vi "UnitTest-Initialize.vi"(8 "error in":errorcluster, 11 "Config IN":T2={"TableLogger"=enum."CSV Logger", "DB File Path"=path "C:/FD/Test.csv", "DB Backup Config"={"Directory"=path "C:/LogAnyLVdata", "UTC Time Format"=FALSE, "On Launch"=TRUE, "Interval (Hours)"=100.0, "Size Multiples (Bytes)"=24}}) -> (0 "error out":errorcluster, 2 "LV Data":T1={"Numeric Data"=1, "Float Data"=1.0, "String Data"="This is string", "Enum Data"=enum."Enum Item 2", "Array Data"=[1234, 2345, 3456, 4567]}, 3 "Config OUT":T2={"TableLogger"=enum."SQLite Logger", "DB File Path"=path "DB.db", "DB Backup Config"={"Directory"=path "DB/Backup", "UTC Time Format"=FALSE, "On Launch"=FALSE, "Interval (Hours)"=100.0, "Size Multiples (Bytes)"=24}})   [LabVIEW 2014]
uses:
  TableLogger_Actor/TableLoggerConfig.ctl
  TableLogger_Actor/TableLoggerTypes.ctl
  TableLogger_Actor/TableLoggerBackupConfig.ctl
  TableLogger_Actor/TableLoggerDataCluster.ctl
  <userlib>/_OpenG.lib/file/file.llb/Strip Path - Traditional__ogtk.vi
  <userlib>/_OpenG.lib/file/file.llb/File Exists - Scalar__ogtk.vi
  <userlib>/_OpenG.lib/file/file.llb/Build Path - Traditional__ogtk.vi
  TableLogger_Actor/TableLogger_Actor.lvlib
panel:
  # "Connector Pane"
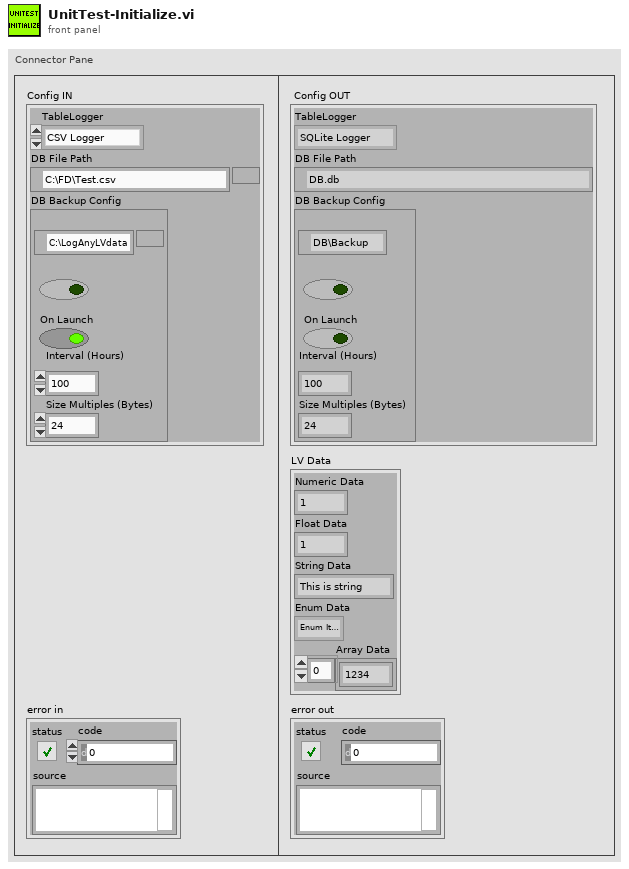
[diagram p1: front panel]
types:
  T1 = typedef "TableLogger_Actor.lvlib/TableLoggerDataCluster.ctl" = cluster{"Numeric Data":i32, "Float Data":dbl, "String Data":string, "Enum Data":enum16{"Enum Item 1", "Enum Item 2"}, "Array Data":i32[]}
  T2 = typedef "TableLogger_Actor.lvlib/TableLoggerConfig.ctl" = cluster{"TableLogger":T3, "DB File Path":path, "DB Backup Config":T4}
  T3 = typedef "TableLogger_Actor.lvlib/TableLoggerTypes.ctl" = enum16{"CSV Logger", "SQLite Logger"}
  T4 = typedef "TableLogger_Actor.lvlib/TableLoggerBackupConfig.ctl" = cluster{"Directory":path, "UTC Time Format":bool, "On Launch":bool, "Interval (Hours)":dbl, "Size Multiples (Bytes)":i32}
  T5 = enum16{"open", "replace", "create", "open or create", "replace or create", "replace or create with confirmation"}
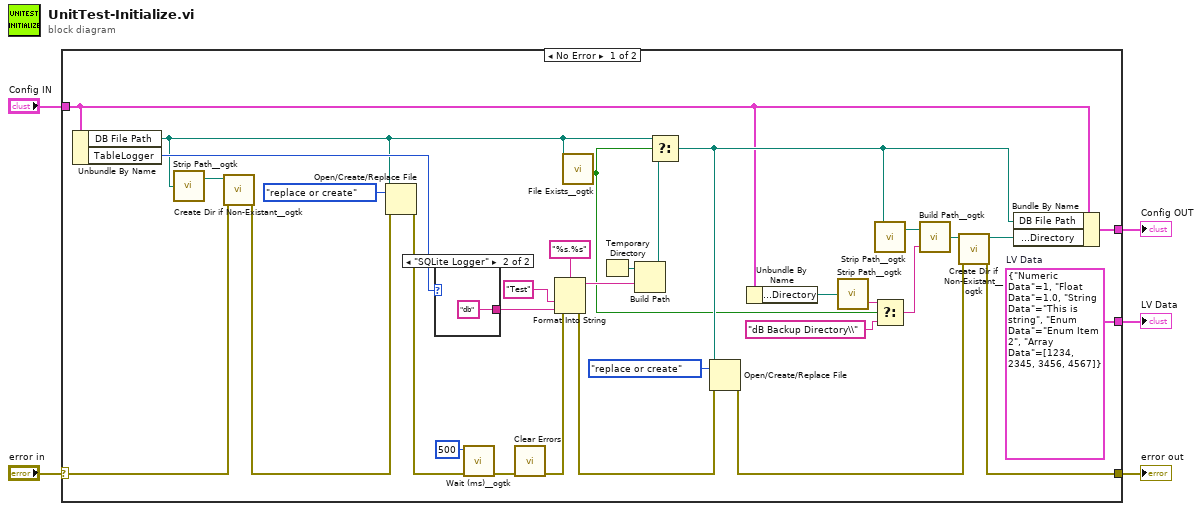
[diagram p0: block diagram]
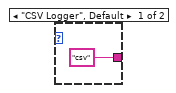
[diagram p2: hidden frame]
diagram:
  n1 = case shown="No Error" "error in" {
    selector: "error in" -> [w8 w41]
    tunnel: [w26 w41] -> w4
    tunnel: "Config IN" -> [w13 w40]
    tunnel: [w34 w40] -> w2
    tunnel: [w6 _] -> w1
    frame No Error {
      w6 = T1 {"Numeric Data"=1, "Float Data"=1.0, "String Data"="This is string", "Enum Data"=enum."Enum Item 2", "Array Data"=[1234, 2345, 3456, 4567]}  # LV Data
      n2 = Unbundle By Name(w13) -> ("DB File Path"=w10:path, "TableLogger"=w33:T3)
      n3 = call-poly <userlib>:"Strip Path__ogtk.vi"("path"=w10) -> ("stripped path"=w9:path)  [unwired: 1 out]
      n4 = call <userlib>:"Create Dir if Non-Existant__ogtk.vi"("error in (no error)"=w8, "Directory Path"=w9) -> ("error out"=w7:errorcluster)  [unwired: 7 in, 2 out]
      n5 = Open/Create/Replace File(file path (use dialog)=w10, error in=w7, operation (0:open)=T5."replace or create") -> (error out=w12:errorcluster)  [unwired: 3 in, 2 out]
      n6 = case shown="\"SQLite Logger\"" w33 {
        tunnel: ["csv" ("format string") "db" ("format string")] -> w32
        frame "CSV Logger", Default {
        }
        frame "SQLite Logger" {
        }
      }
      n7 = call <userlib>:"Wait (ms)__ogtk.vi"("error in (no error)"=w12, "milliseconds to wait"=u32 500) -> ("error out"=w21:errorcluster)  [unwired: 8 in, 1 out]
      n8 = call <vilib>:"Clear Errors.vi"("error in (no error)"=w21) -> ("error out"=w11:errorcluster)  [unwired: 5 in, 1 out]
      n9 = Format Into String(format string="%s.%s", error in=w11, "Test" ("input 1"), w32) -> (resulting string=w35:string, error out=w19:errorcluster)  [unwired: 1 in]
      n10 = call-poly <userlib>:"File Exists__ogtk.vi"("file path"=w10) -> ("exists"=w18:bool)  [unwired: 6 in, 1 out]
      n11 = Temporary Directory() -> (w37:path)
      n12 = Build Path(base path=w37, name or relative path=w35) -> (appended path=w30:path)
      n13 = Select(t=w10, s=w18, f=w30) -> (s? t:f=w25:path)
      n14 = Open/Create/Replace File(file path (use dialog)=w25, error in=w19, operation (0:open)=T5."replace or create") -> (error out=w24:errorcluster)  [unwired: 3 in, 2 out]
      n15 = Unbundle By Name(w13) -> ("DB Backup Config.Directory"=w14:path)
      n16 = call-poly <userlib>:"Strip Path__ogtk.vi"("path"=w14) -> ("name"=w15:string)  [unwired: 1 out]
      n17 = call-poly <userlib>:"Strip Path__ogtk.vi"("path"=w25) -> ("stripped path"=w29:path)  [unwired: 1 out]
      n18 = Select(t=w15, s=w18, f="dB Backup Directory\\" ("name or relative path")) -> (s? t:f=w16:string)
      n19 = call-poly <userlib>:"Build Path__ogtk.vi"("name or relative path"=w16, "base path"=w29) -> ("appended path"=w28:path)
      n20 = call <userlib>:"Create Dir if Non-Existant__ogtk.vi"("error in (no error)"=w24, "Directory Path"=w28) -> ("error out"=w26:errorcluster, "dup Directory Path"=w27:path)  [unwired: 7 in, 1 out]
      n21 = Bundle By Name(cluster=w13, "DB File Path"=w25, "DB Backup Config.Directory"=w27) -> (w34:T2)
    }
    frame Error {
    }
  }
  "error out" <- w4
  "Config OUT" <- w2
  "LV Data" <- w1
